vi "TalkPort.vi"(7 "error constant":errorcluster, 8 "StopThread":bool, 9 "OutString":string, 10 "Port":u16) -> (0 "error out":errorcluster, 1 "Socket Closed":bool)   [LabVIEW 2022 SP3]
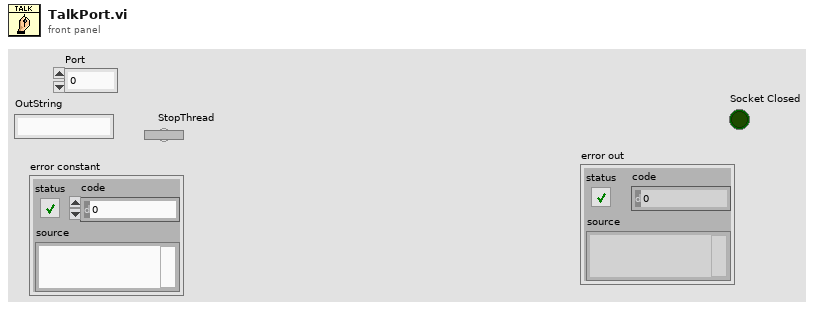
[diagram p1: front panel]
types:
  T1 = enum16{"Standard", "Buffered", "CRLF", "Immediate"}
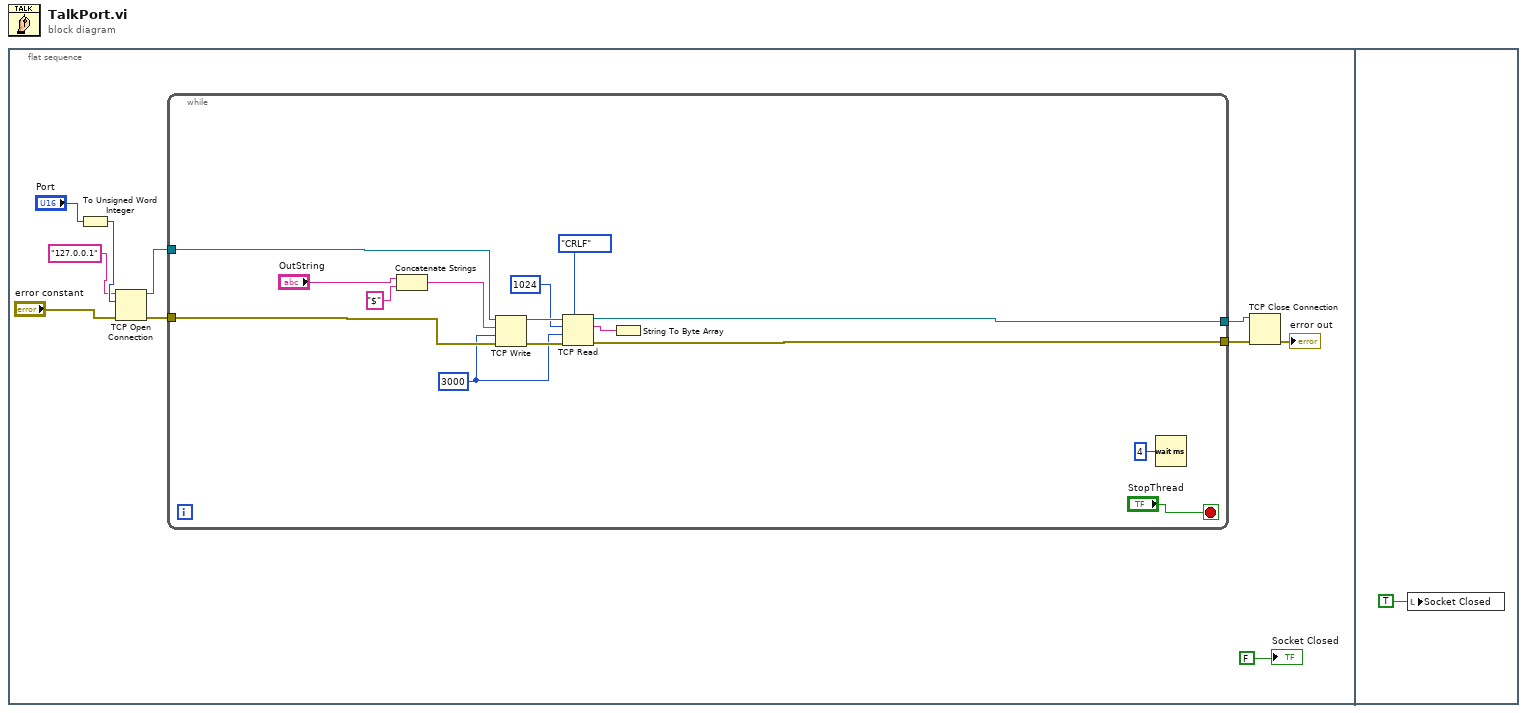
[diagram p0: block diagram]
diagram:
  n1 = flat-sequence {
    frame #0 {
      n2 = To Unsigned Word Integer(number="Port") -> (unsigned 16bit integer=w4:u16)
      n3 = TCP Open Connection(address="127.0.0.1", remote port or service name=w4, error in (no error)="error constant") -> (connection ID=w8:refnum<k5>, error out=w6:errorcluster)  [unwired: 2 in]
      n4 = while {
        tunnel: w6 -> [w24]
        tunnel: [w16] -> w7
        tunnel: w8 -> [w22]
        tunnel: [w15] -> w9
        stop <- "StopThread" stop-if-true
        w19 = 3000 ("timeout ms (25000)")
        n5 = Concatenate Strings("OutString", "$" ("string")) -> (w13:string)
        n6 = TCP Write(connection ID=w22, data in=w13, error in (no error)=w24, 9:w19) -> (connection ID out=w20:refnum<k5>, error out=w21:errorcluster)  [unwired: 1 out]
        n7 = TCP Read(connection ID=w20, bytes to read=1024, error in (no error)=w21, 7:T1."CRLF" ("mode (standard)"), 9:w19) -> (connection ID out=w15:refnum<k5>, data out=w17:string, error out=w16:errorcluster)
        n8 = String To Byte Array(string=w17) -> ()  [unwired: 1 out]
        n9 = Wait (ms)(milliseconds to wait=u32 4) -> ()  [unwired: 1 out]
      }
      n10 = TCP Close Connection(connection ID=w9, error in (no error)=w7) -> (error out=→"error out":errorcluster)  [unwired: 1 in, 1 out]
      "Socket Closed" <- FALSE
    }
    frame #1 {
      n11 = local write "Socket Closed"(TRUE) -> ()
    }
  }
